vi "Get Transfer Buffers.vi"(8 "error in (no error)":errorcluster, 10 "buffer descriptor":T1, 11 "Buffers":T3[](array[typedef])) -> (0 "error out":errorcluster, 3 "Buffer":refnum<class "Buffer.lvclass">)   [LabVIEW 2017, in "DSF Core.lvlib" / "Data Server Thread.lvclass"]
uses:
  Data Server Thread.lvclass
  Buffer/Buffer.lvclass
  C:/Program Files (x86)/National Instruments/LabVIEW 2017/vi.lib/NI/Memory Manager/Classes/Pointer/Pointer.lvclass
  Plugin.ctl
  Buffers/Buffers.lvclass
  Group.ctl
  Transfer/Transfer.lvclass
  DSF Buffer Subset Descriptor.ctl
  Typedefs/DSF Buffer Type.ctl
  <vilib>/NI/Memory Manager/Classes/Pointer/Pointer.lvclass/Pointer.ctl
  <vilib>/NI/Memory Manager/Classes/Pointer/Get Address.vi
  <vilib>/NI/Memory Manager/Classes/Pointer/Encapsulate.vi
  <vilib>/NI/Memory Manager/Classes/Pointer/Check Null Pointer.vi
  <vilib>/NI/Memory Manager/Classes/Pointer/Check Length.vi
  <vilib>/NI/Memory Manager/Classes/Pointer/Set Size.vi
  <vilib>/NI/Memory Manager/Classes/Pointer/Set Address.vi
  <vilib>/NI/Memory Manager/Classes/Pointer/Set Internal.vi
  <vilib>/NI/Memory Manager/Classes/Pointer/Errors.vi
  <vilib>/NI/Memory Manager/Classes/Pointer/Null Pointer.vi
  <vilib>/NI/Memory Manager/Classes/Pointer/Is Null.vi
  <vilib>/NI/Memory Manager/Classes/Pointer/Get Size.vi
  <vilib>/NI/Memory Manager/Classes/Pointer/Check Bounds (Pointer).vi
  <vilib>/NI/Memory Manager/Classes/Pointer/Create Error.vi
  <vilib>/NI/Memory Manager/Classes/Pointer/Out of Bounds.vi
  <vilib>/NI/Memory Manager/Constants/Constants.vi
  <vilib>/NI/Memory Manager/Constants/Library Name.vi
  <vilib>/NI/Memory Manager/Classes/Pointer/Pointer Error Info.vi
  <vilib>/NI/Memory Manager/Constants/Pointer Class Name.vi
  <vilib>/NI/Memory Manager/Classes/Pointer/Write Pointer Size to Error.vi
  <vilib>/NI/Memory Manager/VIs/New Error Cluster.vi
  <vilib>/NI/Memory Manager/VIs/New Error Cluster (512B).vi
  <vilib>/NI/Memory Manager/VIs/Set Error Status.vi
  <vilib>/NI/Memory Manager/VIs/Set Error Code.vi
  <vilib>/NI/Memory Manager/VIs/Set Error Source.vi
  <vilib>/NI/Memory Manager/VIs/Write String to Source.vi
  <vilib>/NI/Memory Manager/VIs/Write Numeric to Source.vi
  <vilib>/NI/Memory Manager/VIs/Write Numeric Scalar to Source (Base10 U64).vi
  DSF Core.lvlib
  <vilib>/NI/Memory Manager/Classes/Pointer/Pointer.lvclass
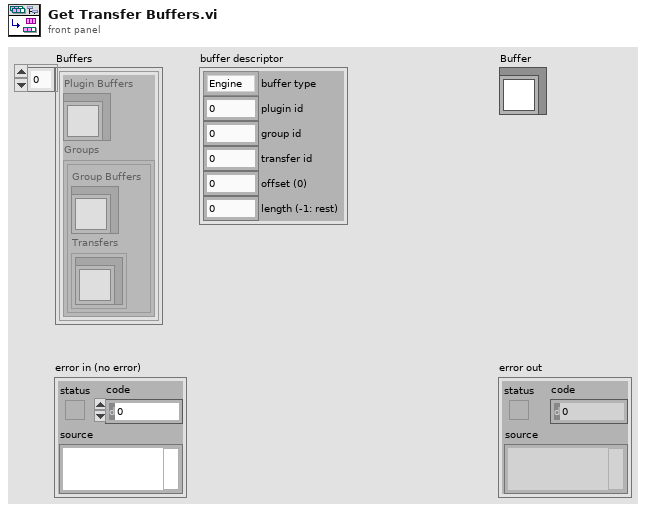
[diagram p1: front panel]
types:
  T1 = typedef "DSF Core.lvlib/DSF Buffer Subset Descriptor.ctl" = cluster{"buffer type":T2, "plugin id":i32, "group id":i32, "transfer id":i32, "offset (0)":u64, "length (-1: rest)":i64}
  T2 = typedef "DSF Core.lvlib/DSF Buffer Type.ctl" = enum16{"Engine", "String"}
  T3 = typedef "DSF Core.lvlib/Data Server Thread.lvclass/Plugin.ctl" = cluster{"Plugin Buffers":refnum<class "Buffers.lvclass">, "Groups":T4[]}
  T4 = typedef "DSF Core.lvlib/Data Server Thread.lvclass/Group.ctl" = cluster{"Group Buffers":refnum<class "Buffers.lvclass">, "Transfers":refnum<class "Transfer.lvclass">[]}
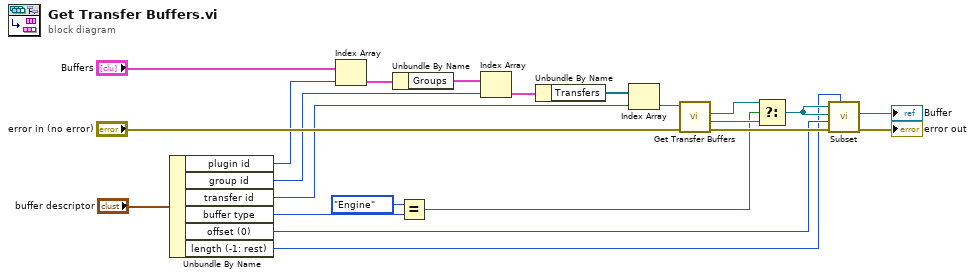
[diagram p0: block diagram]
diagram:
  n1 = Unbundle By Name("buffer descriptor") -> ("plugin id"=w10:i32, "group id"=w9:i32, "transfer id"=w8:i32, "buffer type"=w12:T2, "offset (0)"=w13:u64, "length (-1: rest)"=w4:i64)
  n2 = Index Array(array="Buffers", index=w10) -> (element=w21:T3)
  n3 = Unbundle By Name(w21) -> ("Groups"=w20:T4[])
  n4 = Equal?(x=DSF_Buffer_Type."Engine" ("y"), y=w12) -> (x = y?=w3:bool)
  n5 = Index Array(array=w20, index=w9) -> (element=w19:T4)
  n6 = Unbundle By Name(w19) -> ("Transfers"=w18:refnum<class "Transfer.lvclass">[])
  n7 = Index Array(array=w18, index=w8) -> (element=w17:refnum<class "Transfer.lvclass">)
  n8 = call "Get Transfer Buffers.vi"("error in (no error)"="error in (no error)", "Transfer in"=w17) -> ("error out"=w22:errorcluster, "string Buffer"=w7:refnum<class "Buffer.lvclass">, "engine Buffer"=w6:refnum<class "Buffer.lvclass">)  [unwired: 6 in, 1 out]
  n9 = Select(t=w6, s=w3, f=w7) -> (s? t:f=w5:refnum<class "Buffer.lvclass">)
  n10 = call <vilib>:"Subset.vi"("length (-1: rest)"=w4, "error in (no error)"=w22, "offset (0)"=w13, "subset Pointer type"=w5, "base Pointer in"=w5) -> ("error out"=→"error out":errorcluster, "subset Pointer"=→"Buffer":refnum<class "Buffer.lvclass">)  [unwired: 3 in, 2 out]
